vi "DeQueueMain.vi"(0 "object in":refnum<class "Application.lvclass">=refnum, 2 "timeout in ms (-1)":i32=-1, 5 "error in (no error)":errorcluster) -> (11 "# elements in queue":i32, 14 "object out":refnum<class "Application.lvclass">, 16 "Message":string, 17 "Message Data":variant=variant(errorcluster {"status"=TRUE, "code"=1, "source"="MainTemplate.vi<ERR>\nThe invalid message string \"\" was received in the Message Handling Loop.\n\n\n<b>Complete call chain:</b>\r\n     MainTemplate.vi"}), 19 "error out":errorcluster)   [LabVIEW 2021, in "Application.lvclass"]
uses:
  Application.lvclass
  Hamamatsu_class/Hamamatsu.lvclass
  AD2_SDK_class/AD2_SDK.lvclass
  Valve_class/Valve.lvclass
  Ismatec_class/Ismatec.lvclass
  ExperimentSeries_class/ExperimentSeries.lvclass
  CetoniPump_class/CetoniPump.lvclass
  Prior_Zmotor_class/Prior_Zmotor.lvclass
  ExperimentSeries2_class/ExperimentSeries2.lvclass
  Application.lvclass/Application.ctl
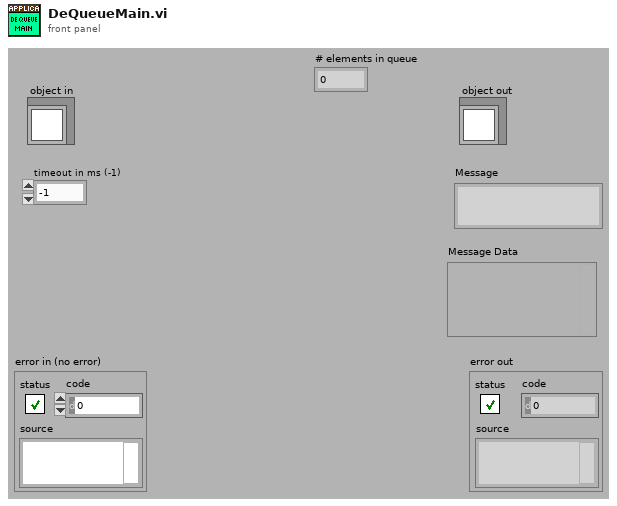
[diagram p1: front panel]
types:
  T1 = cluster{"Message":string, "Message Data":variant}
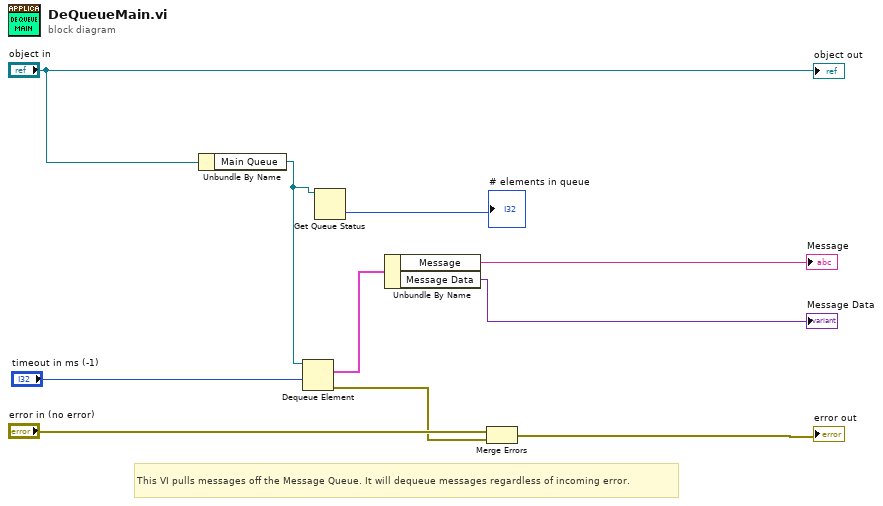
[diagram p0: block diagram]
diagram:
  # "This VI pulls messages off the Message Queue. It will dequeue messages regardless of incoming error."
  n1 = Unbundle By Name("object in") -> ("Main Queue"=w2:refnum<queue>)
  n2 = Dequeue Element(queue=w2, timeout in ms (-1)="timeout in ms (-1)") -> (element=w4:T1, error out=w3:errorcluster)  [unwired: 1 in, 2 out]
  n3 = Get Queue Status(queue=w2) -> (# elements in queue=→"# elements in queue":i32)  [unwired: 2 in, 7 out]
  n4 = Unbundle By Name(w4) -> ("Message"=→"Message":string, "Message Data"=→"Message Data":variant)
  n5 = Merge Errors("error in (no error)", w3) -> (→"error out":errorcluster)
  "object out" <- "object in"
